vi "Get Allocated.vi"(11 "Pointer in":refnum<class "Pointer.lvclass">) -> (2 "allocated":bool, 3 "Pointer out":refnum<class "Pointer.lvclass">)   [LabVIEW 2016, in "Memory Manager.lvlib" / "Pointer.lvclass"]
uses:
  Pointer.lvclass
  Pointer.lvclass/Pointer.ctl
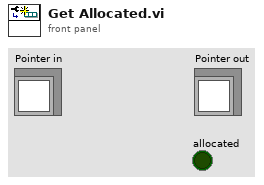
[diagram p1: front panel]
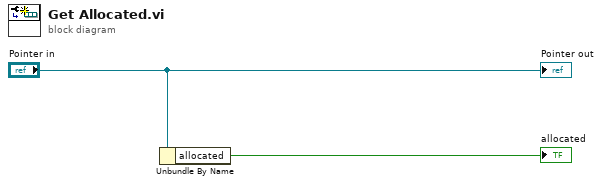
[diagram p0: block diagram]
diagram:
  n1 = Unbundle By Name("Pointer in") -> ("allocated"=→"allocated":bool)
  "Pointer out" <- "Pointer in"
